vi "Q*Q.vi"(2 "quaternion B":dbl[](array[numeric]), 3 "quaternion A":dbl[](array[numeric])) -> (0 "BxA":dbl[](array[numeric]), 1 "AxB":dbl[](array[numeric]))   [LabVIEW 2024]
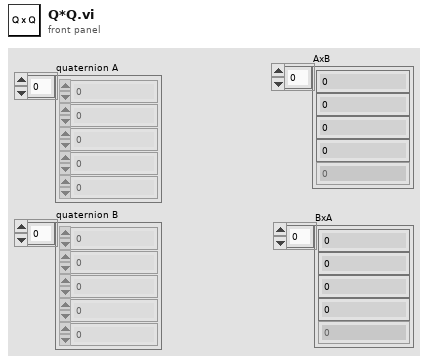
[diagram p1: front panel]
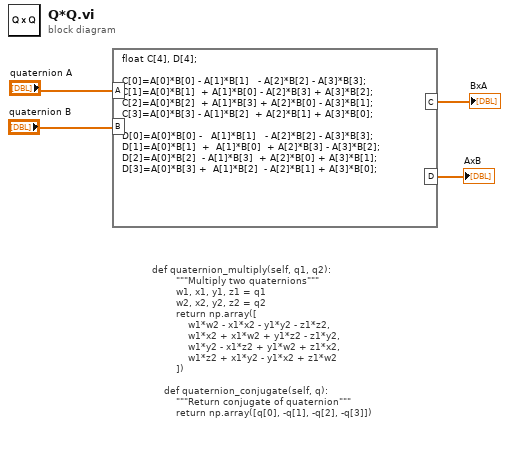
[diagram p0: block diagram]
diagram:
  # "def quaternion_multiply(self, q1, q2):\n        \"\"\"Multiply two quaternions\"\"\"\n        w1, x1, y1, z1 = q1\n        w2, x2, y2, z2 = q2\n        return np.array([\n            w1*w2 - x1*x2 - y1*y2 - z1*z2,\n            w1*x2 + x1*w2 + y1*z2 - z1*y2,\n            w1*y2 - x1*z2 + y1*w2 + z1*x2,\n            w1*z2 + x1*y2 - y1*x2 + z1*w2\n        ])\n\n    def quaternion_conjugate(self, q):\n        \"\"\"Return conjugate of quaternion\"\"\"\n        return np.array([q[0], -q[1], -q[2], -q[3]])"
  n1 = formula code="float C[4], D[4];\n\nC[0]=A[0]*B[0] - A[1]*B[1]   - A[2]*B[2] - A[3]*B[3];\nC[1]=A[0]*B[1]  + A[1]*B[0] - A[2]*B[3] + A[3]*B[2];\nC[2]=A[0]*B[2]  + A[1]*B[3] + A[2]*B[0] - A[3]*B[1];\nC[3]=A[0]*B[3] - A[1]*B[2]  + A[2]*B[1] + A[3]*B[0];\n\nD[0]=A[0]*B[0] -   A[1]*B[1]   - A[2]*B[2] - A[3]*B[3];\nD[1]=A[0]*B[1]  +  A[1]*B[0]  + A[2]*B[3] - A[3]*B[2];\nD[2]=A[0]*B[2]  - A[1]*B[3]  + A[2]*B[0] + A[3]*B[1];\nD[3]=A[0]*B[3] +  A[1]*B[2]  - A[2]*B[1] + A[3]*B[0];"("A"="quaternion A", "B"="quaternion B") -> ("C"=→"BxA":dbl[], "D"=→"AxB":dbl[])
